vi "User Access Level FGV.vi"(8 "错误输入":cluster{"状态":bool, "代码":i32, "源":string}, 10 "用户名":string) -> (0 "错误输出":cluster{"状态":bool, "代码":i32, "源":string}, 1 "用户级别":string)   [LabVIEW 2012]
doc: "该FGV中保存了当前登录用户的访问级别，可执行以下方法：\n\n1. <B>读取用户访问级别文件：</B> 读取一个制表符分隔的文本文件，其中包含用户命和相应的访问级别。\n2. <B>设置当前访问级别：</B> 为输入的用户名设置访问级别。\n3. <B>获取当前访问级别：</B> 返回当前用户的访问级别。"
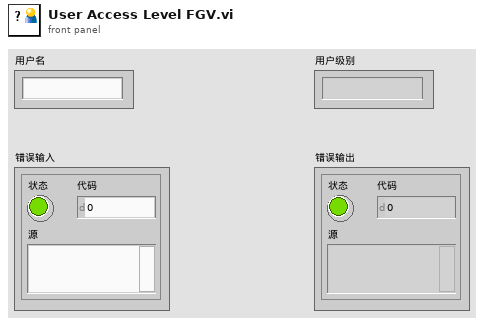
[diagram p1: front panel]
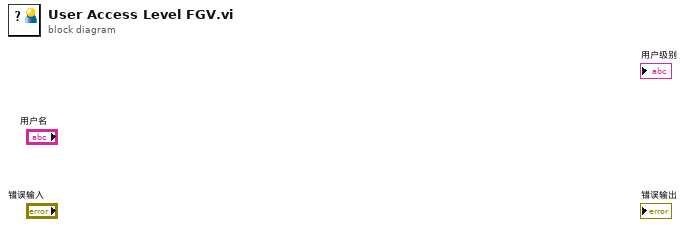
[diagram p0: block diagram]
diagram:
